vi "Kepco DC IDN Parser.vi"(0 "IDN Query":string) -> (4 "Manufacturer":string, 6 "Model":string, 8 "Model #":string, 10 "Firmware Version":string, 14 "Calibrated On":string, 15 "Serial Number":string)   [LabVIEW 2020]
uses:
  Match Regular Expression.xnode
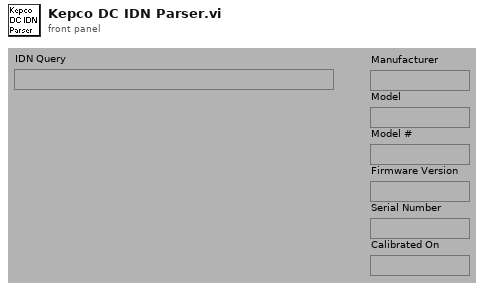
[diagram p1: front panel]
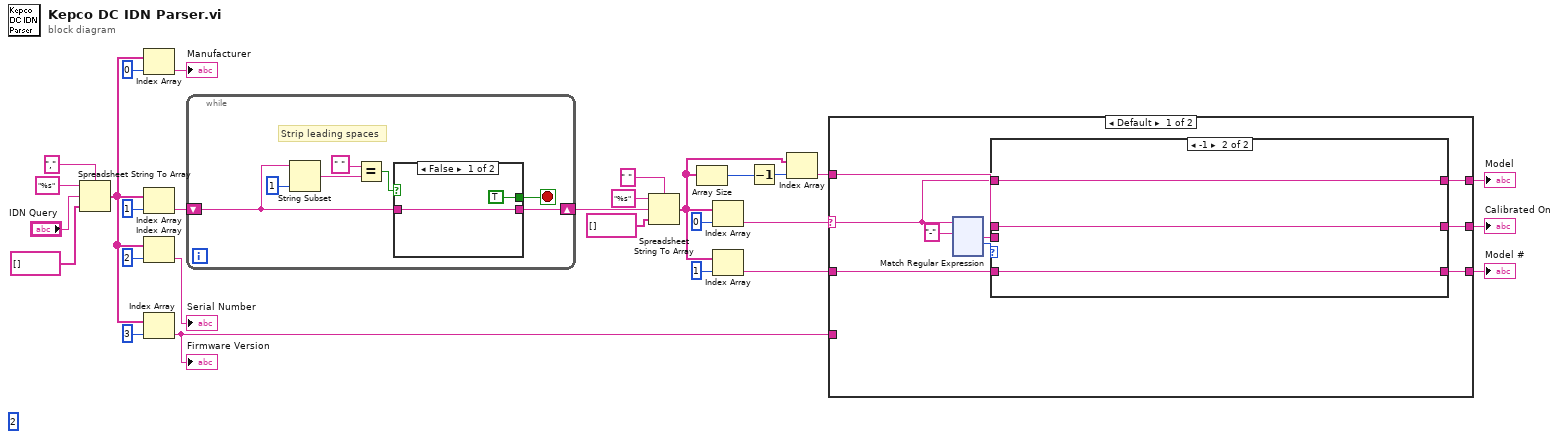
[diagram p0: block diagram]
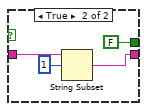
[diagram p2: hidden frame]
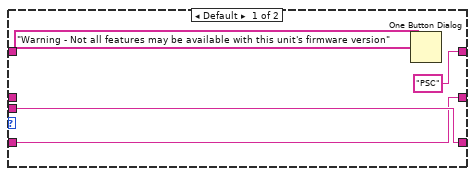
[diagram p3: hidden frame]
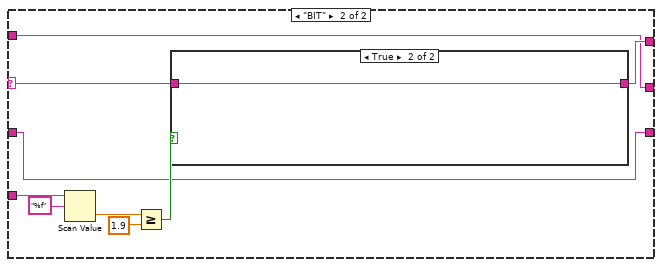
[diagram p4: hidden frame]
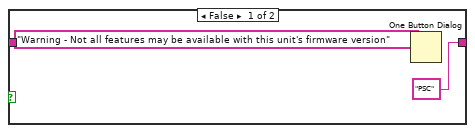
[diagram p5: hidden frame]
diagram:
  (unwired) 2
  n1 = Spreadsheet String To Array(delimiter (Tab)=",", format string="%s", spreadsheet string="IDN Query", array type (2D Dbl)=string[] []) -> (array=w18:string[])
  n2 = Index Array(array=w18, index=0) -> (element=→"Manufacturer":string)
  n3 = Index Array(array=w18, index=1) -> (element=w2:string)
  n4 = Index Array(array=w18, index=2) -> (element=→"Serial Number":string)
  n5 = Index Array(array=w18, index=3) -> (element=w11:string)
  "Firmware Version" <- w11
  n6 = while {
    shift-right: [w30] -> w1
    shift-left: w2 -> [w32]
    stop <- w29 stop-if-true
    # "Strip leading spaces"
    n7 = String Subset(string=w32, length (rest)=1 ("length (rest)")) -> (substring=w34:string)  [unwired: 1 in]
    n8 = Equal?(x=" ", y=w34) -> (x = y?=w31:bool)
    n9 = case shown="False" w31 {
      tunnel: w32 -> [w37 w41]
      tunnel: [w37 w39] -> w30
      tunnel: [TRUE FALSE] -> w29
      frame False {
      }
      frame True {
        n10 = String Subset(string=w41, offset (0)=1) -> (substring=w39:string)  [unwired: 1 in]
      }
    }
  }
  n11 = Spreadsheet String To Array(delimiter (Tab)=" ", format string="%s", spreadsheet string=w1, array type (2D Dbl)=string[] []) -> (array=w5:string[])
  n12 = Array Size(array=w5) -> (size(s)=w4:i32)
  n13 = Index Array(array=w5, index=0) -> (element=w12:string)
  n14 = Index Array(array=w5, index=1) -> (element=w9:string)
  n15 = Decrement(x=w4) -> (x-1=w3:i32)
  n16 = Index Array(array=w5, index=w3) -> (element=w7:string)
  n17 = case shown="Default" w12 {
    selector: w12 -> [w45 w171]
    tunnel: w11 -> [_ w176]
    tunnel: [w50 w172] -> w10
    tunnel: w9 -> [w47 w169]
    tunnel: [w49 w169] -> w8
    tunnel: w7 -> [w46 w170]
    tunnel: [w48 w170] -> w6
    frame Default {
      n18 = xnode "Match Regular Expression"("input string"=w45, "regular expression"="-") -> ("after match"=w42:string, "offset past match"=w43:i32)  [unwired: 2 in, 5 out]
      n19 = case shown="-1" w43 {
        tunnel: w45 -> [_ w168]
        tunnel: ["PSC" w168] -> w50
        tunnel: [w165 w167] -> w49
        tunnel: [w163 w166] -> w48
        tunnel: w47 -> [w163 w167]
        tunnel: w46 -> [_ w166]
        tunnel: w42 -> [w165 _]
        frame Default {
          n20 = One Button Dialog(message="Warning - Not all features may be available with this unit's firmware version") -> ()  [unwired: 2 out]
        }
        frame -1 {
        }
      }
    }
    frame "BIT" {
      n21 = Scan Value(string=w176, format string="%f") -> (value=w177:dbl)  [unwired: 2 out]
      n22 = Greater Or Equal?(x=w177, y=1.9) -> (x >= y?=w174:bool)
      n23 = case shown="True" w174 {
        tunnel: ["PSC" w180] -> w172
        tunnel: w171 -> [_ w180]
        frame False {
          n24 = One Button Dialog(message="Warning - Not all features may be available with this unit's firmware version") -> ()  [unwired: 2 out]
        }
        frame True {
        }
      }
    }
  }
  "Model #" <- w8
  "Model" <- w10
  "Calibrated On" <- w6
